vi "Skew_Image.vi"(0 "[IN] Source Image U16":u16[][](array[numeric]), 1 "[IN] X = Array cols":i32, 2 "[IN] Y = Array rows":i32, 3 "[IN] Share Angle":u16 max=89 step=1, 4 "[IN] Calculation mode":enum16{"Single core", "2x cores", "4x cores"}(ring)) -> (6 "[OUT] Skewed Image":u16[][](array[numeric]))   [LabVIEW 2020]
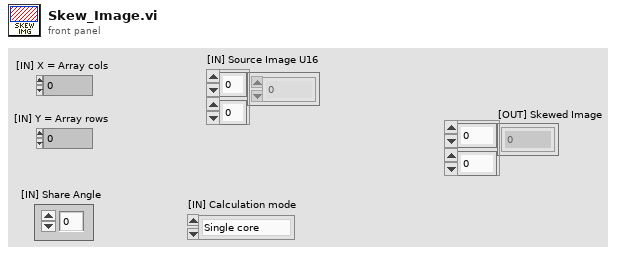
[diagram p1: front panel]
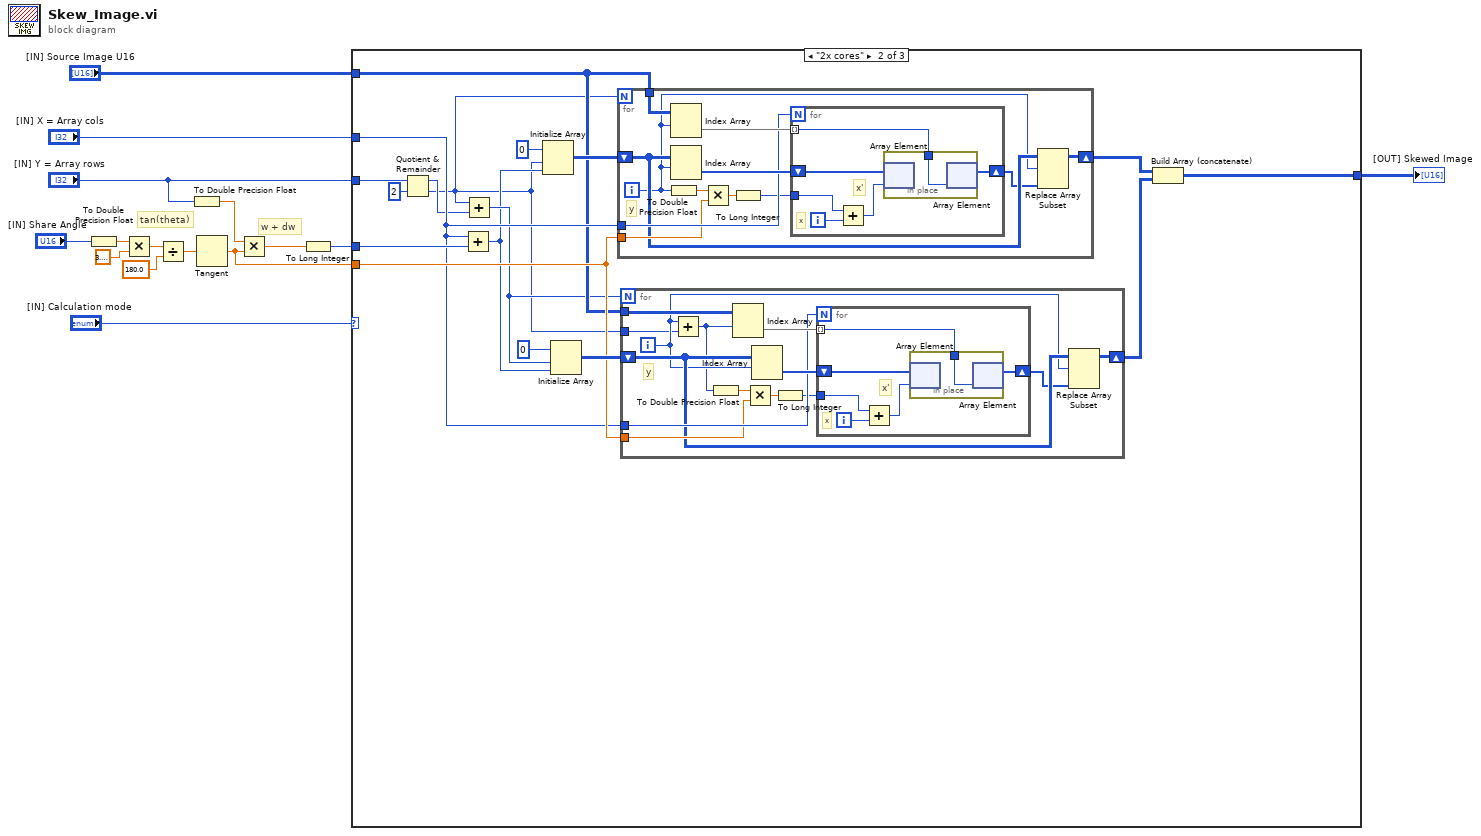
[diagram p0: block diagram]
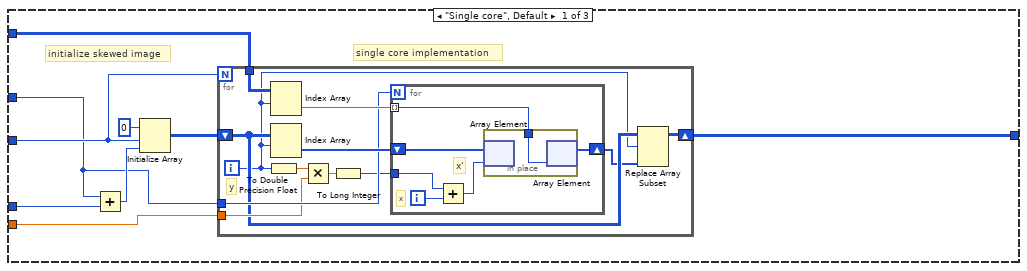
[diagram p2: hidden frame]
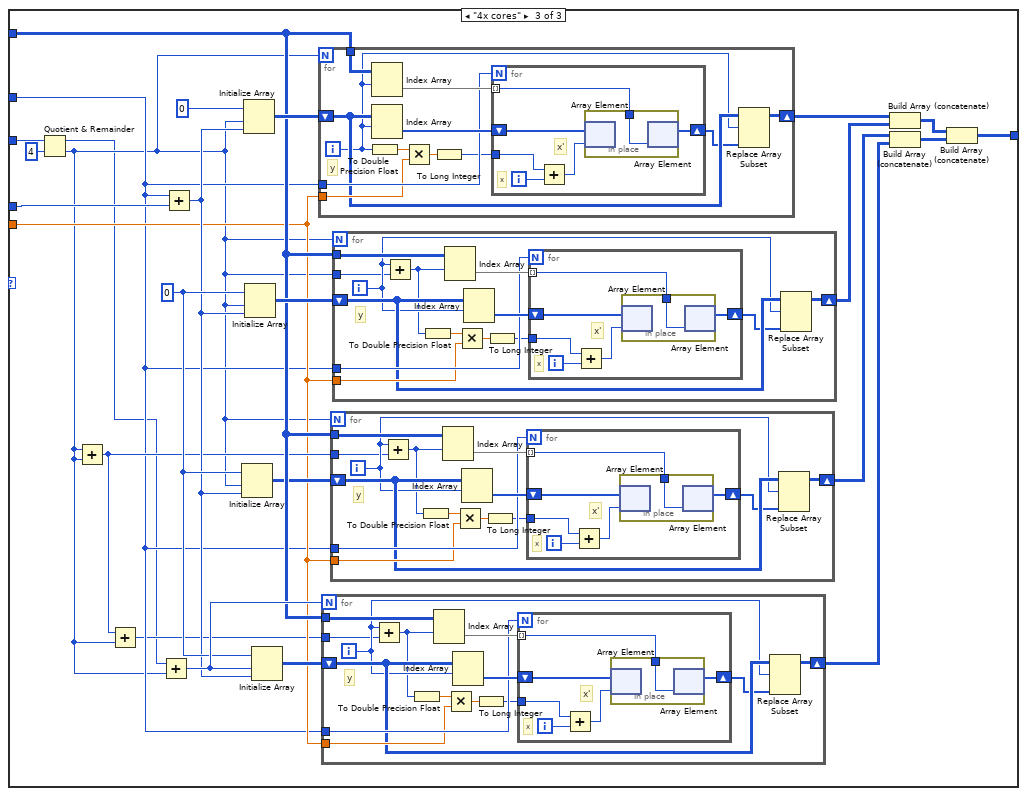
[diagram p3: hidden frame]
diagram:
  # "w + dw"
  # "tan(theta)"
  n1 = To Double Precision Float(number="[IN] Share Angle") -> (double precision float=w15:dbl)
  n2 = Multiply(x=w15, y=3.141592653589793) -> (x*y=w14:dbl)
  n3 = Divide(x=w14, y=180.0) -> (x/y=w12:dbl)
  n4 = To Double Precision Float(number="[IN] Y = Array rows") -> (double precision float=w6:dbl)
  n5 = Tangent(1:w12) -> (0:w10:dbl)
  n6 = Multiply(x=w6, y=w10) -> (x*y=w9:dbl)
  n7 = To Long Integer(number=w9) -> (32bit integer=w11:i32)
  n8 = case shown="\"2x cores\"" "[IN] Calculation mode" {
    tunnel: w11 -> [w23 w58 w120]
    tunnel: w10 -> [w18 w55 w112]
    tunnel: "[IN] Source Image U16" -> [w19 w53 w117]
    tunnel: "[IN] X = Array cols" -> [w16 w54 w111]
    tunnel: "[IN] Y = Array rows" -> [w21 w48 w119]
    tunnel: [w20 w44 w101] -> w3
    frame "Single core", Default {
      # "single core implementation"
      # "initialize skewed image"
      n9 = Add(x=w16, y=w23) -> (x+y=w22:i32)
      n10 = Initialize Array(u16 0, w21, w22) -> (w17:u16[][])
      n11 = for {
        N: w21 -> [_]
        shift-right: [w27] -> w20
        shift-left: w17 -> [w28]
        tunnel: w19 -> [w35]
        tunnel: w16 -> [w33]
        tunnel: w18 -> [w31]
        i -> [w26]
        # "y"
        n12 = To Double Precision Float(number=w26) -> (double precision float=w32:dbl)
        n13 = Index Array(array=w35, index (row)=w26) -> (element=w34:u16[])  [unwired: 1 in]
        n14 = Index Array(array=w28, index (row)=w26) -> (element=w36:u16[])  [unwired: 1 in]
        n15 = Multiply(x=w32, y=w31) -> (x*y=w30:dbl)
        n16 = To Long Integer(number=w30) -> (32bit integer=w29:i32)
        n17 = for {
          N: w33 -> [_]
          shift-right: [w38] -> w25
          shift-left: w36 -> [w40]
          tunnel: w34 -> [w37] mode=indexing
          tunnel: w29 -> [w41]
          i -> [w42]
          # "x'"
          # "x"
          n18 = Add(x=w41, y=w42) -> (x+y=w39:i32)
          n19 = in-place {
            in-place-border: w37 -> [w43]
            n20 = in-place-array #1(w40, w39) -> ()  [unwired: 1 out]
            n21 = in-place-array #1(w43) -> (w38:u16[])  [unwired: 1 out]
          }
        }
        n22 = Replace Array Subset(array=w28, new element=w25, index (row)=w26) -> (w27:u16[][])  [unwired: 1 in]
      }
    }
    frame "2x cores" {
      n23 = Quotient & Remainder(x=w48, y=2) -> (x-y*floor(x/y)=w52:i32, floor(x/y)=w47:i32)
      n24 = Add(x=w54, y=w58) -> (x+y=w49:i32)
      n25 = Add(x=w47, y=w52) -> (x+y=w51:i32)
      n26 = Initialize Array(u16 0, w47, w49) -> (w57:u16[][])
      n27 = Initialize Array(u16 0, w51, w49) -> (w56:u16[][])
      n28 = for {
        N: w47 -> [_]
        shift-right: [w84] -> w46
        shift-left: w57 -> [w85]
        tunnel: w53 -> [w92]
        tunnel: w54 -> [w90]
        tunnel: w55 -> [w88]
        i -> [w83]
        # "y"
        n29 = To Double Precision Float(number=w83) -> (double precision float=w89:dbl)
        n30 = Index Array(array=w92, index (row)=w83) -> (element=w91:u16[])  [unwired: 1 in]
        n31 = Index Array(array=w85, index (row)=w83) -> (element=w93:u16[])  [unwired: 1 in]
        n32 = Multiply(x=w89, y=w88) -> (x*y=w87:dbl)
        n33 = To Long Integer(number=w87) -> (32bit integer=w86:i32)
        n34 = for {
          N: w90 -> [_]
          shift-right: [w95] -> w82
          shift-left: w93 -> [w97]
          tunnel: w91 -> [w94] mode=indexing
          tunnel: w86 -> [w98]
          i -> [w99]
          # "x'"
          # "x"
          n35 = Add(x=w98, y=w99) -> (x+y=w96:i32)
          n36 = in-place {
            in-place-border: w94 -> [w100]
            n37 = in-place-array #2(w97, w96) -> ()  [unwired: 1 out]
            n38 = in-place-array #2(w100) -> (w95:u16[])  [unwired: 1 out]
          }
        }
        n39 = Replace Array Subset(array=w85, new element=w82, index (row)=w83) -> (w84:u16[][])  [unwired: 1 in]
      }
      n40 = for {
        N: w51 -> [_]
        shift-right: [w65] -> w45
        shift-left: w56 -> [w66]
        tunnel: w53 -> [w73]
        tunnel: w54 -> [w71]
        tunnel: w55 -> [w69]
        tunnel: w47 -> [w62]
        i -> [w63]
        # "y"
        n41 = Add(x=w63, y=w62) -> (x+y=w61:i32)
        n42 = To Double Precision Float(number=w61) -> (double precision float=w70:dbl)
        n43 = Index Array(array=w73, index (row)=w61) -> (element=w72:u16[])  [unwired: 1 in]
        n44 = Multiply(x=w70, y=w69) -> (x*y=w68:dbl)
        n45 = Index Array(array=w66, index (row)=w63) -> (element=w74:u16[])  [unwired: 1 in]
        n46 = To Long Integer(number=w68) -> (32bit integer=w67:i32)
        n47 = for {
          N: w71 -> [_]
          shift-right: [w76] -> w64
          shift-left: w74 -> [w78]
          tunnel: w72 -> [w75] mode=indexing
          tunnel: w67 -> [w79]
          i -> [w80]
          # "x'"
          # "x"
          n48 = Add(x=w79, y=w80) -> (x+y=w77:i32)
          n49 = in-place {
            in-place-border: w75 -> [w81]
            n50 = in-place-array #3(w78, w77) -> ()  [unwired: 1 out]
            n51 = in-place-array #3(w81) -> (w76:u16[])  [unwired: 1 out]
          }
        }
        n52 = Replace Array Subset(array=w66, new element=w64, index (row)=w63) -> (w65:u16[][])  [unwired: 1 in]
      }
      n53 = Build Array (concatenate)(w46, w45) -> (w44:u16[][])
    }
    frame "4x cores" {
      w116 = u16 0
      n54 = Quotient & Remainder(x=w119, y=4) -> (x-y*floor(x/y)=w108:i32, floor(x/y)=w109:i32)
      n55 = Add(x=w109, y=w109) -> (x+y=w113:i32)
      n56 = Add(x=w113, y=w109) -> (x+y=w110:i32)
      n57 = Add(x=w108, y=w109) -> (x+y=w121:i32)
      n58 = Add(x=w111, y=w120) -> (x+y=w115:i32)
      n59 = Initialize Array(w116, w109, w115) -> (w114:u16[][])
      n60 = Initialize Array(u16 0, w109, w115) -> (w123:u16[][])
      n61 = Initialize Array(w116, w109, w115) -> (w118:u16[][])
      n62 = Initialize Array(w116, w121, w115) -> (w122:u16[][])
      n63 = for {
        N: w109 -> [_]
        shift-right: [w191] -> w107
        shift-left: w123 -> [w192]
        tunnel: w117 -> [w199]
        tunnel: w111 -> [w197]
        tunnel: w112 -> [w195]
        i -> [w190]
        # "y"
        n64 = To Double Precision Float(number=w190) -> (double precision float=w196:dbl)
        n65 = Index Array(array=w199, index (row)=w190) -> (element=w198:u16[])  [unwired: 1 in]
        n66 = Index Array(array=w192, index (row)=w190) -> (element=w200:u16[])  [unwired: 1 in]
        n67 = Multiply(x=w196, y=w195) -> (x*y=w194:dbl)
        n68 = To Long Integer(number=w194) -> (32bit integer=w193:i32)
        n69 = for {
          N: w197 -> [_]
          shift-right: [w202] -> w189
          shift-left: w200 -> [w204]
          tunnel: w198 -> [w201] mode=indexing
          tunnel: w193 -> [w205]
          i -> [w206]
          # "x'"
          # "x"
          n70 = Add(x=w205, y=w206) -> (x+y=w203:i32)
          n71 = in-place {
            in-place-border: w201 -> [w207]
            n72 = in-place-array #4(w204, w203) -> ()  [unwired: 1 out]
            n73 = in-place-array #4(w207) -> (w202:u16[])  [unwired: 1 out]
          }
        }
        n74 = Replace Array Subset(array=w192, new element=w189, index (row)=w190) -> (w191:u16[][])  [unwired: 1 in]
      }
      n75 = for {
        N: w121 -> [_]
        shift-right: [w172] -> w104
        shift-left: w122 -> [w173]
        tunnel: w117 -> [w180]
        tunnel: w111 -> [w178]
        tunnel: w112 -> [w176]
        tunnel: w110 -> [w169]
        i -> [w170]
        # "y"
        n76 = Add(x=w170, y=w169) -> (x+y=w168:i32)
        n77 = To Double Precision Float(number=w168) -> (double precision float=w177:dbl)
        n78 = Index Array(array=w180, index (row)=w168) -> (element=w179:u16[])  [unwired: 1 in]
        n79 = Multiply(x=w177, y=w176) -> (x*y=w175:dbl)
        n80 = Index Array(array=w173, index (row)=w170) -> (element=w181:u16[])  [unwired: 1 in]
        n81 = To Long Integer(number=w175) -> (32bit integer=w174:i32)
        n82 = for {
          N: w178 -> [_]
          shift-right: [w183] -> w171
          shift-left: w181 -> [w185]
          tunnel: w179 -> [w182] mode=indexing
          tunnel: w174 -> [w186]
          i -> [w187]
          # "x'"
          # "x"
          n83 = Add(x=w186, y=w187) -> (x+y=w184:i32)
          n84 = in-place {
            in-place-border: w182 -> [w188]
            n85 = in-place-array #5(w185, w184) -> ()  [unwired: 1 out]
            n86 = in-place-array #5(w188) -> (w183:u16[])  [unwired: 1 out]
          }
        }
        n87 = Replace Array Subset(array=w173, new element=w171, index (row)=w170) -> (w172:u16[][])  [unwired: 1 in]
      }
      n88 = for {
        N: w109 -> [_]
        shift-right: [w130] -> w105
        shift-left: w114 -> [w131]
        tunnel: w117 -> [w138]
        tunnel: w111 -> [w136]
        tunnel: w112 -> [w134]
        tunnel: w113 -> [w127]
        i -> [w128]
        # "y"
        n89 = Add(x=w128, y=w127) -> (x+y=w126:i32)
        n90 = To Double Precision Float(number=w126) -> (double precision float=w135:dbl)
        n91 = Index Array(array=w138, index (row)=w126) -> (element=w137:u16[])  [unwired: 1 in]
        n92 = Multiply(x=w135, y=w134) -> (x*y=w133:dbl)
        n93 = Index Array(array=w131, index (row)=w128) -> (element=w139:u16[])  [unwired: 1 in]
        n94 = To Long Integer(number=w133) -> (32bit integer=w132:i32)
        n95 = for {
          N: w136 -> [_]
          shift-right: [w141] -> w129
          shift-left: w139 -> [w143]
          tunnel: w137 -> [w140] mode=indexing
          tunnel: w132 -> [w144]
          i -> [w145]
          # "x'"
          # "x"
          n96 = Add(x=w144, y=w145) -> (x+y=w142:i32)
          n97 = in-place {
            in-place-border: w140 -> [w146]
            n98 = in-place-array #6(w143, w142) -> ()  [unwired: 1 out]
            n99 = in-place-array #6(w146) -> (w141:u16[])  [unwired: 1 out]
          }
        }
        n100 = Replace Array Subset(array=w131, new element=w129, index (row)=w128) -> (w130:u16[][])  [unwired: 1 in]
      }
      n101 = for {
        N: w109 -> [_]
        shift-right: [w151] -> w106
        shift-left: w118 -> [w152]
        tunnel: w117 -> [w159]
        tunnel: w111 -> [w157]
        tunnel: w112 -> [w155]
        tunnel: w109 -> [w148]
        i -> [w149]
        # "y"
        n102 = Add(x=w149, y=w148) -> (x+y=w147:i32)
        n103 = To Double Precision Float(number=w147) -> (double precision float=w156:dbl)
        n104 = Index Array(array=w159, index (row)=w147) -> (element=w158:u16[])  [unwired: 1 in]
        n105 = Multiply(x=w156, y=w155) -> (x*y=w154:dbl)
        n106 = Index Array(array=w152, index (row)=w149) -> (element=w160:u16[])  [unwired: 1 in]
        n107 = To Long Integer(number=w154) -> (32bit integer=w153:i32)
        n108 = for {
          N: w157 -> [_]
          shift-right: [w162] -> w150
          shift-left: w160 -> [w164]
          tunnel: w158 -> [w161] mode=indexing
          tunnel: w153 -> [w165]
          i -> [w166]
          # "x'"
          # "x"
          n109 = Add(x=w165, y=w166) -> (x+y=w163:i32)
          n110 = in-place {
            in-place-border: w161 -> [w167]
            n111 = in-place-array #7(w164, w163) -> ()  [unwired: 1 out]
            n112 = in-place-array #7(w167) -> (w162:u16[])  [unwired: 1 out]
          }
        }
        n113 = Replace Array Subset(array=w152, new element=w150, index (row)=w149) -> (w151:u16[][])  [unwired: 1 in]
      }
      n114 = Build Array (concatenate)(w107, w106) -> (w103:u16[][])
      n115 = Build Array (concatenate)(w105, w104) -> (w102:u16[][])
      n116 = Build Array (concatenate)(w103, w102) -> (w101:u16[][])
    }
  }
  "[OUT] Skewed Image" <- w3
